vi "Unpack DBL Value.vi"(11 "DBLValueMsg in":refnum<class "DBLValueMsg.lvclass">) -> (2 "Value":dbl, 3 "Name":string)   [LabVIEW 2015, in "ActorAutoRegistration.lvlib" / "DBLValueMsg.lvclass"]
uses:
  DBLValueMsg.lvclass
  DBLValueMsg.lvclass/DBLValueMsg.ctl
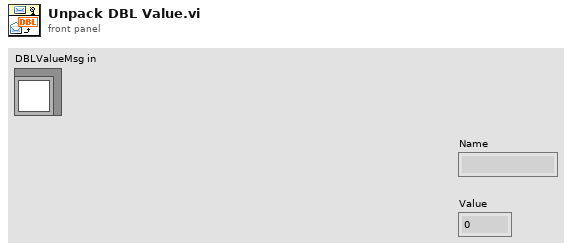
[diagram p1: front panel]
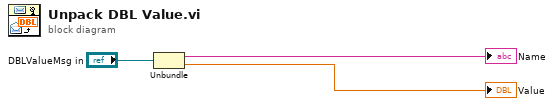
[diagram p0: block diagram]
diagram:
  n1 = Unbundle("DBLValueMsg in") -> (→"Name":string, →"Value":dbl)
